vi "crea vector theta cero r.vi"(9 "q máximo":dbl, 10 "q mínimo":dbl, 11 "Resolución":dbl) -> (1 "Vector resolución (r)":dbl[](array[numeric]), 2 "Tamaño (r)":i32, 3 "q0r":dbl[](array[numeric]))   [LabVIEW 2013]
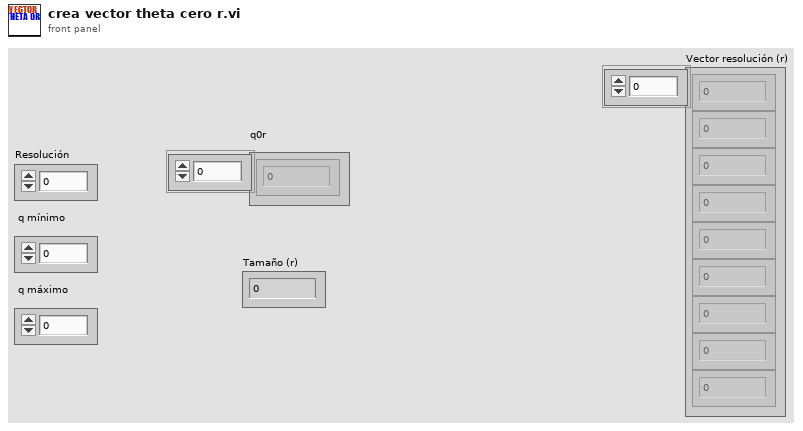
[diagram p1: front panel]
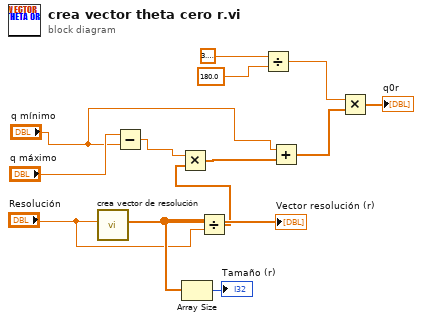
[diagram p0: block diagram]
diagram:
  n1 = call "crea vector de resolución.vi"("Resolución"="Resolución") -> ("Vector resolución (r)"=w12:dbl[])  [unwired: 10 in]
  "Vector resolución (r)" <- w12
  n2 = Subtract(x="q máximo", y="q mínimo") -> (x-y=w10:dbl)
  n3 = Array Size(array=w12) -> (size(s)=→"Tamaño (r)":i32)
  n4 = Divide(x=w12, y="Resolución") -> (x/y=w9:dbl[])
  n5 = Multiply(x=w10, y=w9) -> (x*y=w7:dbl[])
  n6 = Divide(x=3.141592653589793, y=180.0) -> (x/y=w4:dbl)
  n7 = Add(x="q mínimo", y=w7) -> (x+y=w3:dbl[])
  n8 = Multiply(x=w4, y=w3) -> (x*y=→"q0r":dbl[])
